vi "draw to acquire line profile and centroid.vi"() -> ()   [LabVIEW 2014]
uses:
  <vilib>/vision/NI_Vision_Development_Module.lvlib
panel:
  in  "File Path":path
  out "Centroid":cluster{"X Centroid":sgl, "Y Centroid":sgl} {"Y Centroid" format="%.2f"; "X Centroid" format="%.2f"}
  out "混合信号图":cluster{"x0":sgl, "dx":sgl, "Pixels Line":sgl[]}(graph)
  out "Other Parameters":sgl[](array[numeric])
  out "Coordinates":i32[](array[numeric])
  in  "停止":bool
  out "11":T1(plugin-control)
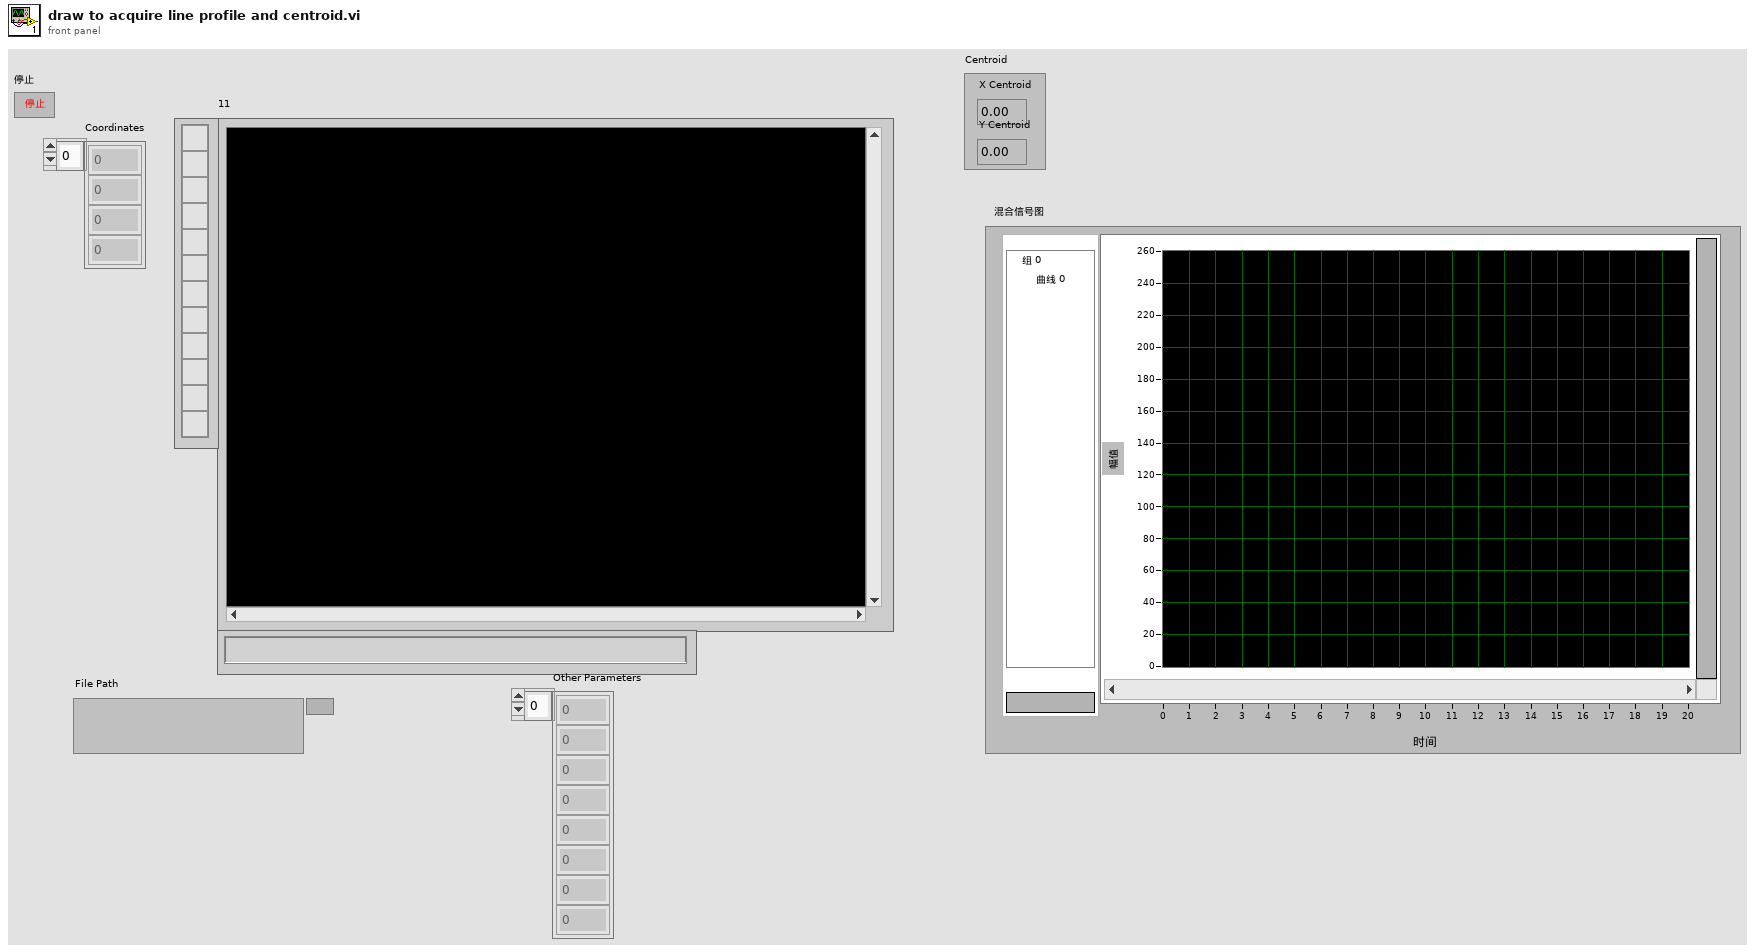
[diagram p1: front panel]
types:
  T1 = typedef "IMAQ Image.ctl" = refnum<image>
  T2 = typedef "Image Type" = u32
  T3 = cluster{"Coordinates[0]":i32, "Coordinates[1]":i32, "Coordinates[2]":i32, "Coordinates[3]":i32, "Coordinates[4]":i32, "Coordinates[5]":i32, "Coordinates[6]":i32, "Coordinates[7]":i32, "Coordinates[8]":i32}
  T4 = cluster{"Coordinates[0]":i32, "Coordinates[1]":i32, "Coordinates[2]":i32, "Coordinates[3]":i32, i32}
  T5 = typedef "ROI Descriptor" = cluster{"Global Rectangle":i32[], "Contours":cluster{"ID":enum32{"External", "Internal"}, "Type":u32, "Coordinates":i32[]}[]}
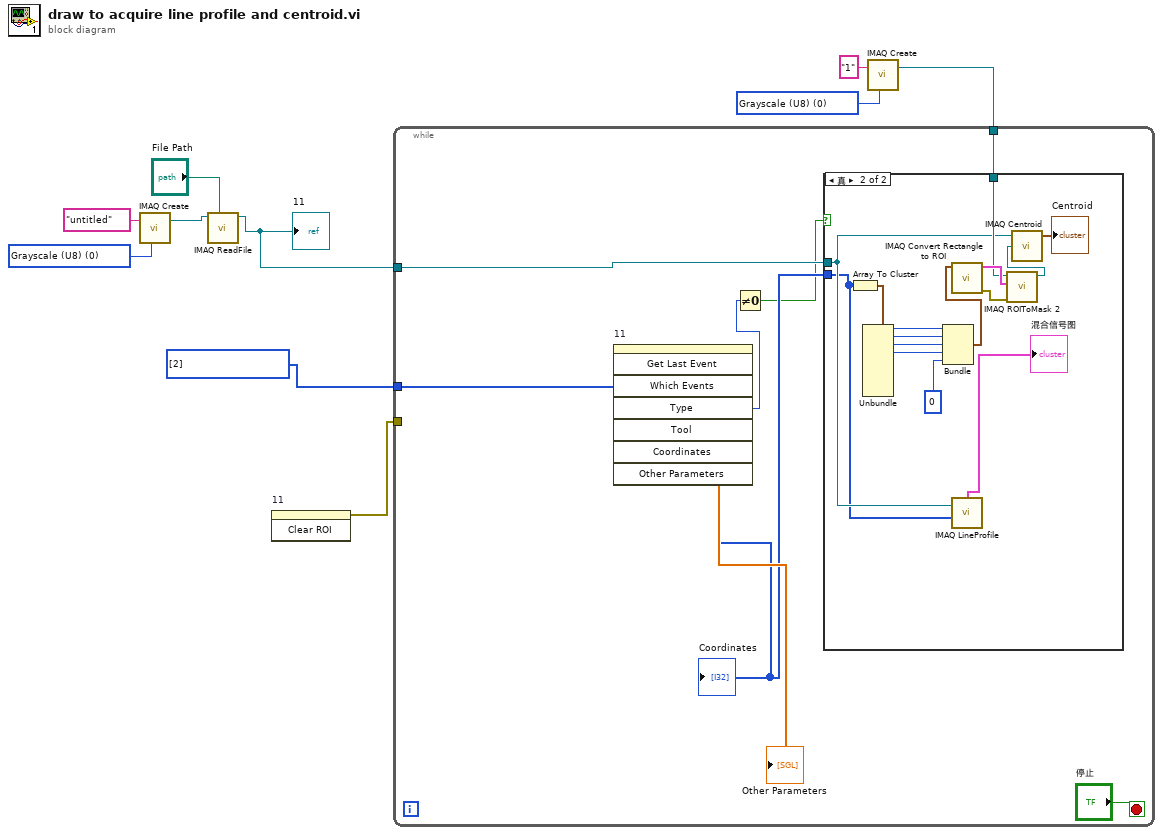
[diagram p0: block diagram]
diagram:
  w3 = T2 0 items=["Grayscale (U8)", "Grayscale (I16)", "Grayscale (SGL)", "Complex (CSG)", "RGB (U32)", "HSL (U32)", "RGB (U64)", "Grayscale (U16)"] ("Image Type")
  w5 = i32[] [2] items=["No Event"=0, "Click Event"=1, "Draw Event"=2, "Size Event"=4, "Scroll Event"=5, "Double Click Event"=8] ("Which Events")
  w8 = T2 0 items=["Grayscale (U8)", "Grayscale (I16)", "Grayscale (SGL)", "Complex (CSG)", "RGB (U32)", "HSL (U32)", "RGB (U64)", "Grayscale (U16)"] ("Image Type")
  n1 = call "IMAQ Create"("Image Name"="untitled", "Image Type"=w8) -> ("New Image"=w7:T1)  [unwired: 3 in, 1 out]
  n2 = call "IMAQ ReadFile"("File Path"="File Path", "Image"=w7) -> ("Image Out"=w6:T1)  [unwired: 5 in, 4 out]
  "11" <- w6
  n3 = invoke on="11" class="ImageControl" method="Clear ROI"() -> (error out=w10:errorcluster)  [unwired: 3 in, 2 out]
  n4 = call "IMAQ Create"("Image Name"="1", "Image Type"=w3) -> ("New Image"=w2:T1)  [unwired: 3 in, 1 out]
  n5 = while {
    tunnel: w10 -> [_]
    tunnel: w6 -> [w16]
    tunnel: w5 -> [w14]
    tunnel: w2 -> [w11]
    stop <- "停止" stop-if-true
    n6 = invoke on="11" class="ImageControl" method="Get Last Event"("Which Events"=w14) -> ("Type"=w13:i32, "Coordinates"=w15:i32[], "Other Parameters"=→"Other Parameters":sgl[])  [unwired: 7 in, 5 out]
    "Coordinates" <- w15
    n7 = Not Equal To 0?(x=w13) -> (x != 0?=w12:bool)
    n8 = case shown="真" w12 {
      tunnel: w16 -> [_ w21]
      tunnel: w15 -> [_ w20]
      tunnel: w11 -> [_ w24]
      frame False {
      }
      frame True {
        n9 = Array To Cluster(array=w20) -> (cluster=w33:T3)
        n10 = Unbundle(w33) -> ("Coordinates[0]"=w32:i32, "Coordinates[1]"=w31:i32, "Coordinates[2]"=w30:i32, "Coordinates[3]"=w29:i32)  [unwired: 5 out]
        n11 = Bundle("Coordinates[0]"=w32, "Coordinates[1]"=w31, "Coordinates[2]"=w30, "Coordinates[3]"=w29, 0) -> (w27:T4)  [unwired: 1 in]
        n12 = call "IMAQ Convert Rectangle to ROI"("Rectangle"=w27) -> ("error out"=w26:errorcluster, "ROI Descriptor"=w25:T5)  [unwired: 8 in]
        n13 = call "IMAQ LineProfile"("Line Coordinates"=w20, "Image"=w21) -> ("Line Graph"=→"混合信号图":cluster{"x0":sgl, "dx":sgl, "Pixels Line":sgl[]})  [unwired: 3 in, 3 out]
        n14 = call "IMAQ ROIToMask 2"("error in (no error)"=w26, "ROI Descriptor"=w25, "Image"=w24) -> ("Image Out"=w23:T1)  [unwired: 6 in, 2 out]
        n15 = call "IMAQ Centroid"("Image Mask"=w23, "Image"=w21) -> ("Centroid"=→"Centroid":cluster{"X Centroid":sgl, "Y Centroid":sgl})  [unwired: 2 in, 1 out]
      }
    }
  }
